vi "CRYASIOGetInputDeviceNames.vi"(10 "Driver Name":string, 11 "error in (no error)":errorcluster) -> (1 "Channel Idx":u32[](array[numeric]), 2 "Output Device Names":string[](array[string]), 3 "error out":errorcluster)   [LabVIEW 2013]
uses:
  CRY_ASIO.dll
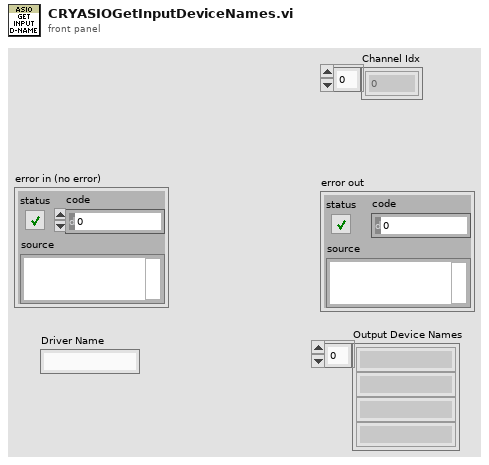
[diagram p1: front panel]
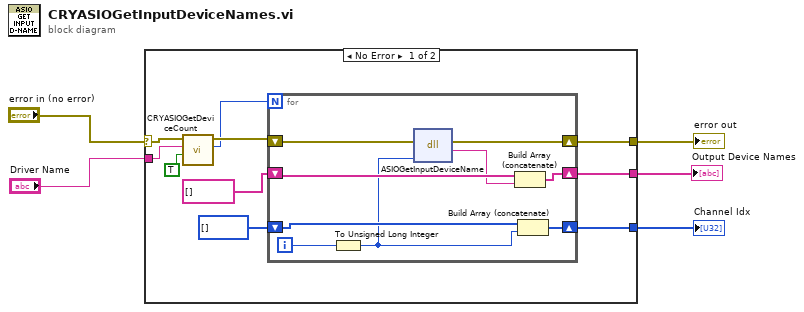
[diagram p0: block diagram]
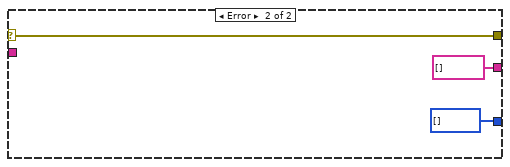
[diagram p2: hidden frame]
diagram:
  n1 = case shown="No Error" "error in (no error)" {
    selector: "error in (no error)" -> [w13 w26]
    tunnel: "Driver Name" -> [w12 _]
    tunnel: [w15 w26] -> w2
    tunnel: [w14 string[] [] ("appended array")] -> w3
    tunnel: [w11 i32[] [] ("appended array")] -> w1
    frame No Error {
      n2 = call "CRYASIOGetDeviceCount.vi"("InOut"=TRUE, "Driver Name"=w12, "error in (no error)"=w13) -> ("Device Count"=w8:u32, "error out"=w9:errorcluster)  [unwired: 7 in]
      n3 = for {
        N: w8 -> [_]
        shift-right: [w23] -> w14
        shift-left: string[] [] ("appended array") -> [w24]
        shift-right: [w19] -> w15
        shift-left: w9 -> [w20]
        shift-right: [w17] -> w11
        shift-left: i32[] [] ("appended array") -> [w18]
        i -> [w22]
        n4 = To Unsigned Long Integer(number=w22) -> (unsigned 32bit integer=w16:u32)
        n5 = dll-call lib="D:/LabView_Project/CRY6181/CRY_ASIO.dll" fn="ASIOGetInputDeviceName"(error in=w20, "devID"=w16) -> (error out=w19:errorcluster, "return type"=w21:string)  [unwired: 3 in, 1 out]
        n6 = Build Array (concatenate)(w24, w21) -> (w23:string[])
        n7 = Build Array (concatenate)(w18, w16) -> (w17:u32[])
      }
    }
    frame Error {
    }
  }
  "Output Device Names" <- w3
  "error out" <- w2
  "Channel Idx" <- w1
